vi "Read Next DBL.vi"(8 "error in (no error)":errorcluster, 11 "object in":refnum<class "CAN IO.lvclass">) -> (0 "error out":errorcluster, 2 "Value Read":dbl, 3 "object out":refnum<class "CAN IO.lvclass">)   [LabVIEW 2013, in "CAN IO.lvclass"]
uses:
  CAN IO.lvclass
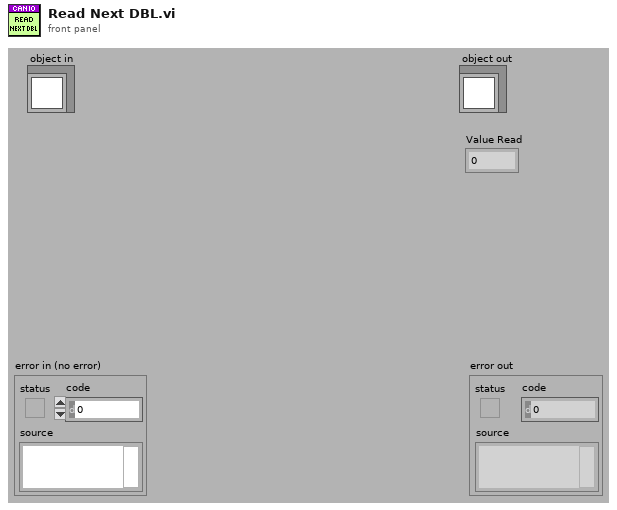
[diagram p1: front panel]
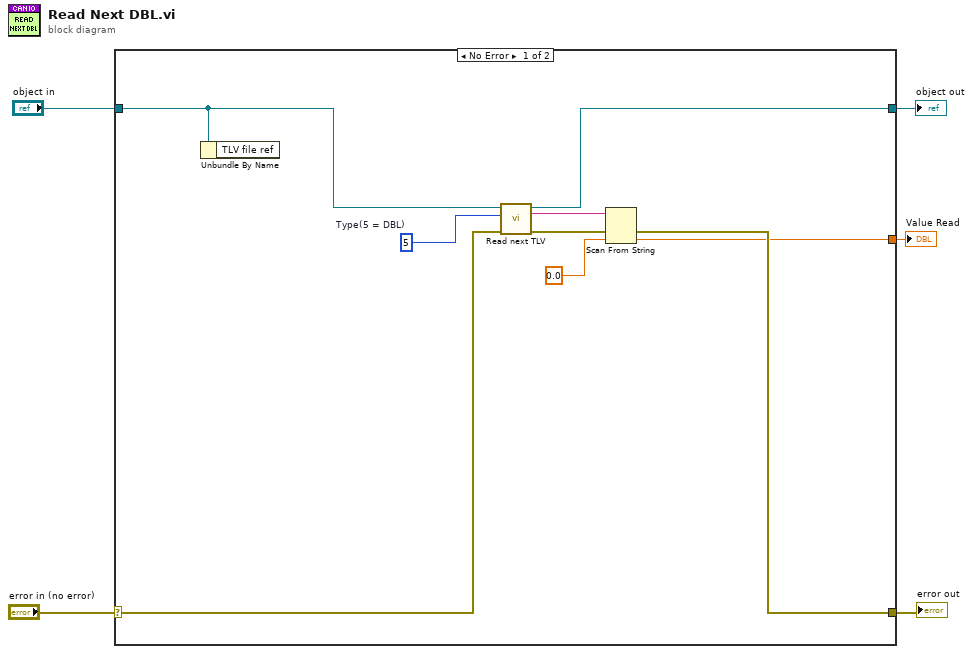
[diagram p0: block diagram]
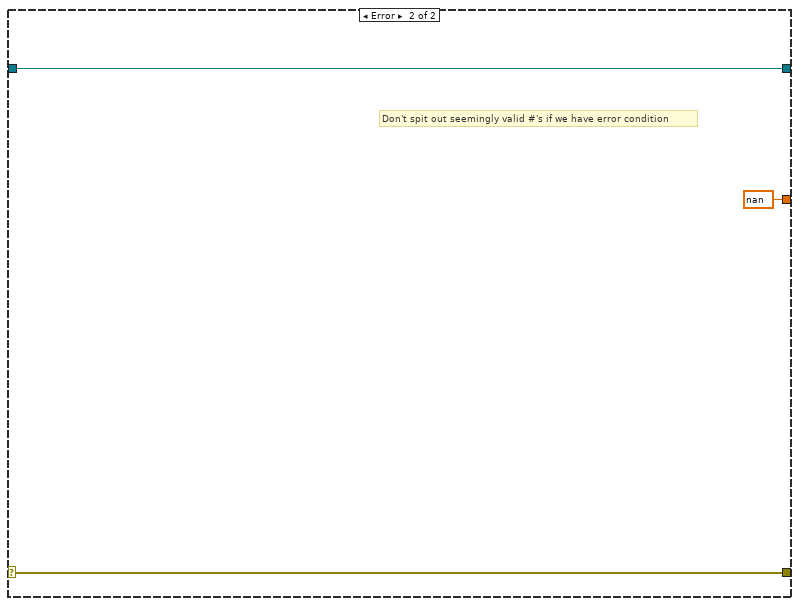
[diagram p2: hidden frame]
diagram:
  n1 = case shown="No Error" "error in (no error)" {
    selector: "error in (no error)" -> [w8 w17]
    tunnel: [w7 w17] -> w4
    tunnel: [w11 w16] -> w2
    tunnel: "object in" -> [w12 w16]
    tunnel: [w6 nan ("default value 1")] -> w1
    frame No Error {
      w14 = u8 5  # Type(5 = DBL)
      n2 = Unbundle By Name(w12) -> ()  [unwired: 1 out]
      n3 = call-dynamic "Read next TLV.vi"("error in (no error)"=w8, "Type(255=next available)"=w14, "object in"=w12) -> ("error out"=w10:errorcluster, "TLV Payload"=w13:string, "object out"=w11:refnum<class "CAN IO.lvclass">)  [unwired: 6 in]
      n4 = Scan From String(input string=w13, error in=w10, default 1=0.0 ("default value 1")) -> (error out=w7:errorcluster, output 1=w6:dbl)  [unwired: 2 in, 2 out]
    }
    frame Error {
      # "Don't spit out seemingly valid #'s if we have error condition"
    }
  }
  "error out" <- w4
  "object out" <- w2
  "Value Read" <- w1
